vi "Find decimal line in console response.vi"(8 "error in (no error)":errorcluster, 11 "Console response in":string) -> (0 "error out":errorcluster, 1 "output decimal line":string, 2 "Decimal Number":i32, 3 "Found decimal line":bool)   [LabVIEW 2024]
uses:
  <vilib>/Utility/error.llb/Trim Whitespace One-Sided.vi
panel:
  out "Line number (0-n)":i32
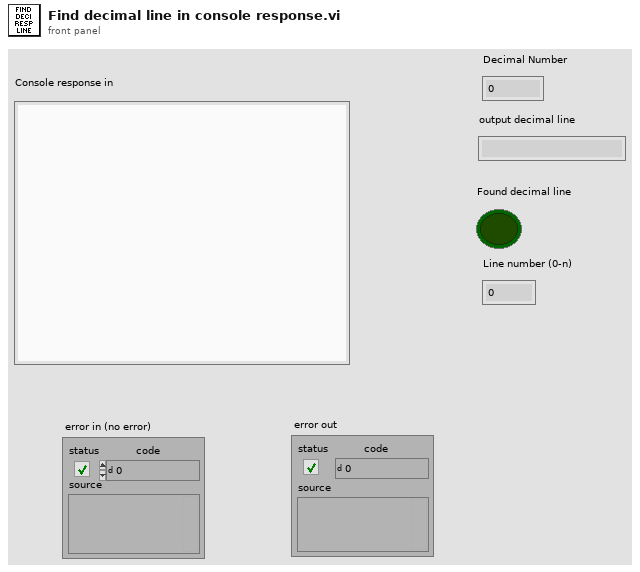
[diagram p1: front panel]
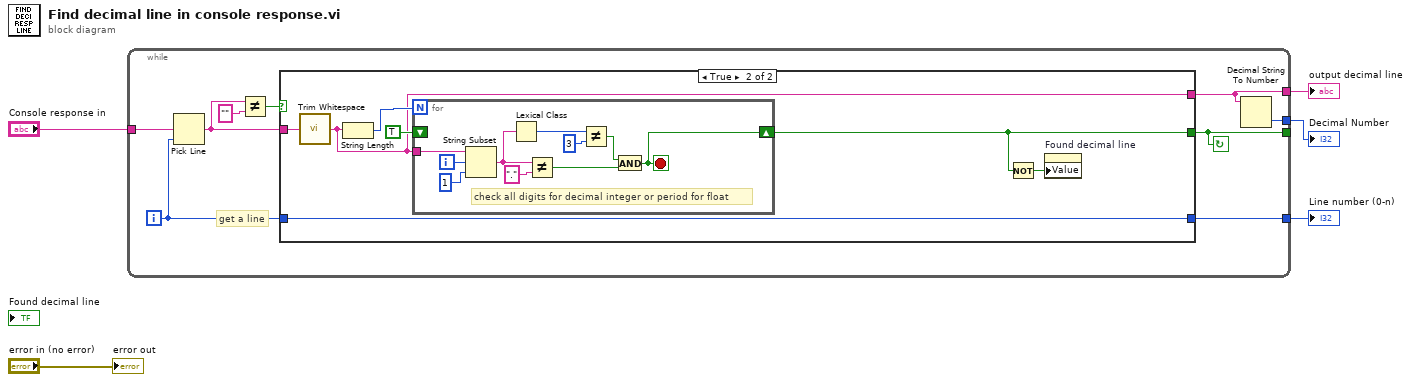
[diagram p0: block diagram]
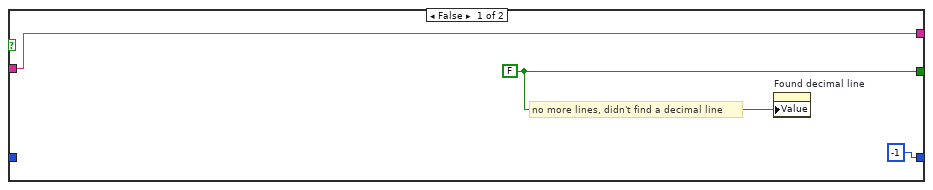
[diagram p2: hidden frame]
diagram:
  n1 = while {
    tunnel: "Console response in" -> [w14]
    tunnel: [w9] -> w3
    tunnel: [w10] -> _
    tunnel: [w8] -> w2
    tunnel: [w7] -> w1
    i -> [w6]
    stop <- w10 continue-if-true
    # "get a line"
    n2 = Pick Line(multi-line string=w14, line index=w6) -> (output string=w11:string)  [unwired: 1 in]
    n3 = Not Equal?(x=w11, y="") -> (x != y?=w12:bool)
    n4 = case shown="True" w12 {
      tunnel: w11 -> [w17 w24]
      tunnel: [w16 w19] -> w10
      tunnel: [w17 w21] -> w9
      tunnel: [-1 w18] -> w7
      tunnel: w6 -> [_ w18]
      frame False {
        w16 = FALSE
        # "no more lines, didn't find a decimal line"
        n5 = property on="Found decimal line" class="Bool (strict)"("Value"=w16) -> ()  [unwired: 2 in, 2 out]
      }
      frame True {
        n6 = call <vilib>:"Trim Whitespace.vi"("string"=w24) -> ("trimmed string"=w21:string)  [unwired: 1 in]
        n7 = String Length(string=w21) -> (length=w23:i32)
        n8 = for {
          N: w23 -> [_]
          shift-right: [w25] -> w19
          shift-left: TRUE -> [_]
          tunnel: w21 -> [w32]
          i -> [w34]
          stop <- w25 stop-if-true
          # "check all digits for decimal integer or period for float"
          n9 = String Subset(string=w32, offset (0)=w34, length (rest)=1 ("length (rest)")) -> (substring=w29:string)
          n10 = Lexical Class(1:w29) -> (0:w31:i16)
          n11 = Not Equal?(x=w29, y=".") -> (x != y?=w26:bool)
          n12 = Not Equal?(x=w31, y=i16 3) -> (x != y?=w27:bool)
          n13 = And(x=w27, y=w26) -> (x .and. y?=w25:bool)
        }
        n14 = Not(x=w19) -> (.not. x?=w20:bool)
        n15 = property on="Found decimal line" class="Bool (strict)"("Value"=w20) -> ()  [unwired: 2 in, 2 out]
      }
    }
    n16 = Decimal String To Number(string=w9) -> (number=w8:i32)  [unwired: 2 in, 1 out]
  }
  "output decimal line" <- w3
  "Decimal Number" <- w2
  "Line number (0-n)" <- w1
  "error out" <- "error in (no error)"
